vi "Interval Timer with Data Storage.vi"() -> ()   [LabVIEW 2011]
panel:
  out "output array 2":dbl[][](array[numeric])
  out "output array":dbl[](array[numeric])
  out "Relative Time":dbl
  out "test":bool
  out "Waveform Chart":cluster{i16, i16}(graph)
  in  "Interval (sec)":dbl=2.0
  in  "Delay (sec)":dbl(knob)=0.20637723542731085 scale=0.0..1.0
  in  "Width (sec)":dbl(knob)=0.500001840510888 scale=0.0..1.0
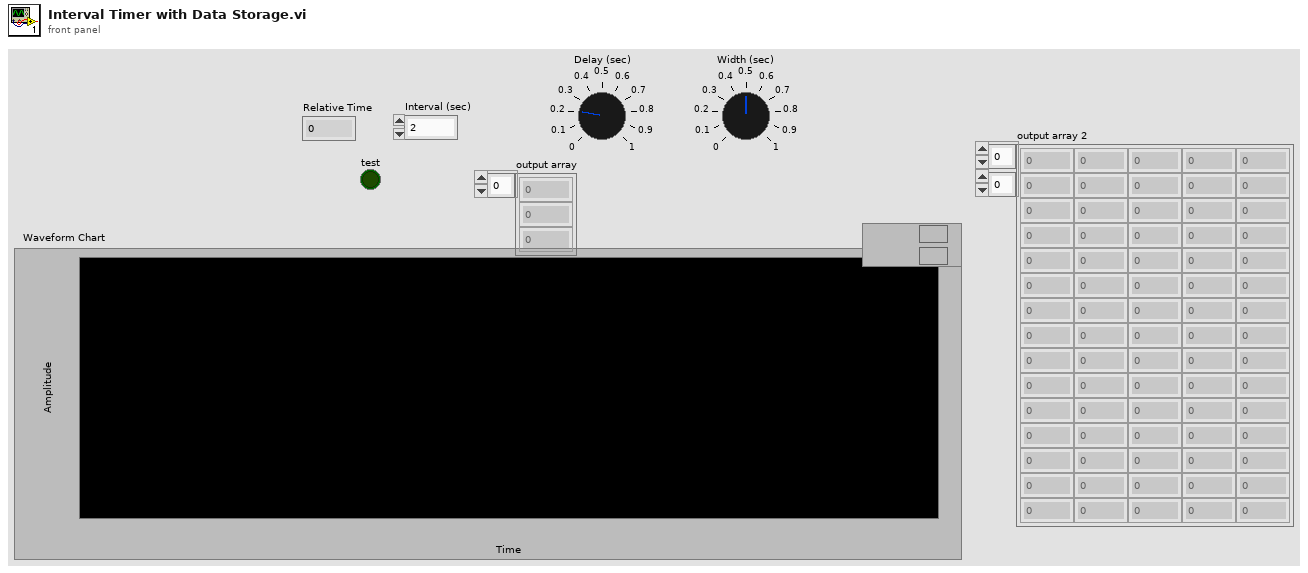
[diagram p1: front panel]
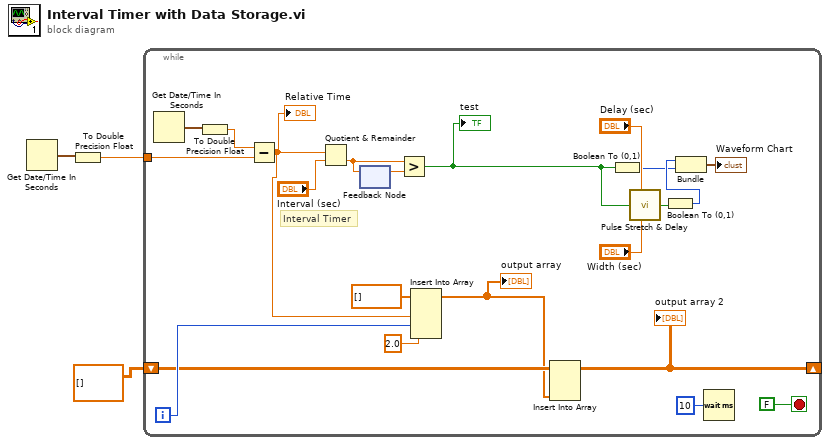
[diagram p0: block diagram]
diagram:
  n1 = Get Date/Time In Seconds() -> (seconds since 1Jan1904=w3:timestamp)
  n2 = To Double Precision Float(number=w3) -> (double precision float=w2:dbl)
  n3 = while {
    tunnel: w2 -> [w23]
    shift-right: [w5] -> _
    shift-left: dbl[][] [] ("array") -> [w6]
    i -> [w7]
    stop <- FALSE stop-if-true
    # "Interval Timer"
    n4 = Get Date/Time In Seconds() -> (seconds since 1Jan1904=w25:timestamp)
    n5 = To Double Precision Float(number=w25) -> (double precision float=w24:dbl)
    n6 = Subtract(x=w24, y=w23) -> (x-y=w9:dbl)
    "Relative Time" <- w9
    n7 = Quotient & Remainder(x=w9, y="Interval (sec)") -> (floor(x/y)=w20:dbl)  [unwired: 1 out]
    n8 = feedback-in #1(w20) -> ()
    n9 = feedback #1() -> (w19:dbl)  [unwired: 1 in]
    n10 = Greater?(x=w20, y=w19) -> (0:w11:bool)
    "test" <- w11
    n11 = Insert Into Array(array=dbl[] [], new element #1=w9, new element #2=w7, new element #3=2.0 ("new element/subarray")) -> (w4:dbl[])  [unwired: 1 in]
    "output array" <- w4
    n12 = Insert Into Array(array=w6, new element=w4) -> (w5:dbl[][])  [unwired: 2 in]
    "output array 2" <- w5
    n13 = Boolean To (0,1)(Boolean=w11) -> (0, 1=w12:i16)
    n14 = call "Pulse Stretch & Delay.vi"("Delay (sec)"="Delay (sec)", "In"=w11, "Width (sec)"="Width (sec)") -> ("Out"=w17:bool)  [unwired: 2 in]
    n15 = Boolean To (0,1)(Boolean=w17) -> (0, 1=w13:i16)
    n16 = Bundle(w13, w12) -> (→"Waveform Chart":cluster{i16, i16})  [unwired: 1 in]
    n17 = Wait (ms)(milliseconds to wait=u32 10) -> ()  [unwired: 1 out]
  }
